vi "Write WorkDir 2.vi"(8 "error in (no error)":errorcluster, 10 "WorkDir":path, 11 "HIJ Vision Application in":refnum<class "HIJ Vision Application.lvclass">) -> (0 "error out":errorcluster, 3 "HIJ Vision Application out":refnum<class "HIJ Vision Application.lvclass">)   [LabVIEW 2020]
uses:
  HIJ Vision Application.lvclass
  HIJ Vision Application.lvclass/HIJ Vision Application.ctl
  C:/Users/AlexK/work/LabVIEW Programme/POLARIS CAM Log Abw und E/Submodules/Viewable Actor/ViewableActor/ViewableActor.lvclass
  C:/Program Files (x86)/National Instruments/LabVIEW 2020/vi.lib/ActorFramework/Actor/Actor.lvclass
  C:/Users/AlexK/work/LabVIEW Programme/POLARIS CAM Log Abw und E/Submodules/HIJ Vision/Application Base Actors/HIJ Vision Application/HIJ Vision Application/HIJ Vision Application.lvclass
  C:/Users/AlexK/work/LabVIEW Programme/POLARIS CAM Log Abw und E/Submodules/HIJ Vision/Analyze/Analyze Actor/IAnalysis/IAnalysis.lvclass
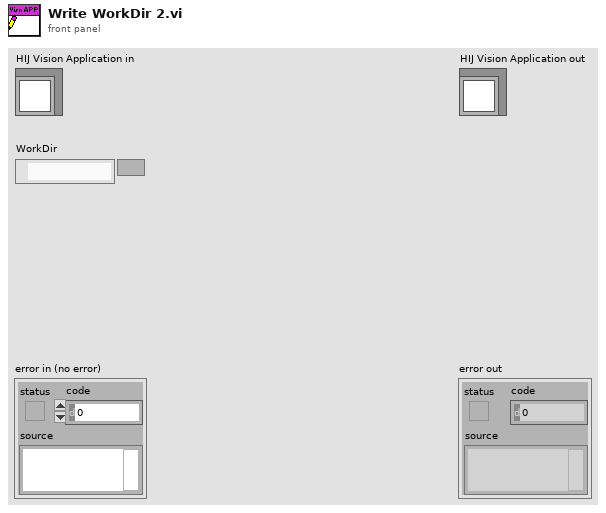
[diagram p1: front panel]
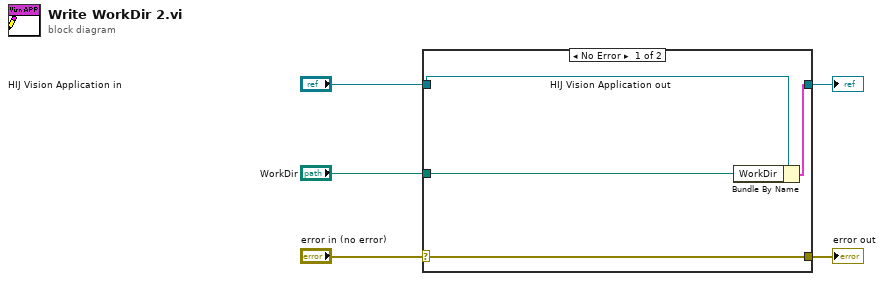
[diagram p0: block diagram]
diagram:
  n1 = case shown="No Error" "error in (no error)" {
    selector: "error in (no error)" -> [w9 w10]
    tunnel: [w9 w10] -> w4
    tunnel: [w7 w11] -> w2
    tunnel: "HIJ Vision Application in" -> [w8 w11]
    tunnel: "WorkDir" -> [w6 _]
    frame No Error {
      n2 = Bundle By Name(cluster=w8, "WorkDir"=w6) -> (w7:cluster{})
    }
    frame Error {
    }
  }
  "error out" <- w4
  "HIJ Vision Application out" <- w2
